vi "will_heading_hit_obstacles.vi"(8 "Distance to check (m)":dbl, 9 "Heading":dbl, 10 "Boat Location":T1 {"North" format="%#_10f"; "East" format="%#_8f"}, 11 "Obstacle array":refnum<class "Obstacle.lvclass">[](array[class])) -> (3 "Will boat hit any obstacles?":bool)   [LabVIEW 2013]
uses:
  Obstacle.lvclass
  Data/TypeDefs/UTM Location.ctl
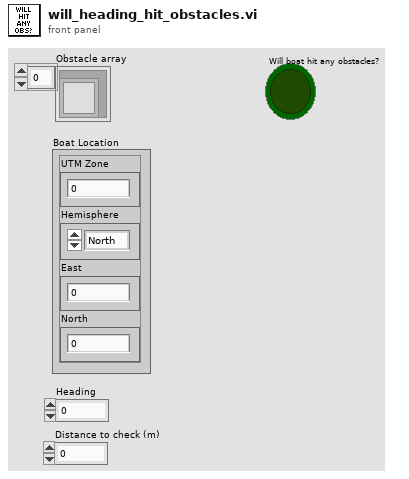
[diagram p1: front panel]
types:
  T1 = typedef "UTM Location.ctl" = cluster{"UTM Zone":dbl, "Hemisphere":enum16{"North", "South"}, "East":dbl, "North":dbl}
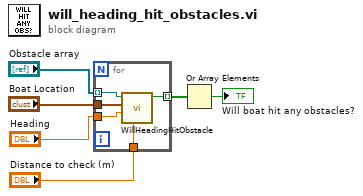
[diagram p0: block diagram]
diagram:
  n1 = for {
    tunnel: "Obstacle array" -> [w11] mode=indexing
    tunnel: [w10] -> w6 mode=indexing
    tunnel: "Boat Location" -> [w9]
    tunnel: "Heading" -> [w8]
    tunnel: "Distance to check (m)" -> [w7]
    n2 = call "WillHeadingHitObstacle.vi"("Distance to check (m)"=w7, "Heading"=w8, "Boat"=w9, "Obstacle.lvclass"=w11) -> ("Any intersecting obstacles?"=w10:bool)  [unwired: 6 in, 1 out]
  }
  n3 = Or Array Elements(Boolean array=w6) -> (logical OR=→"Will boat hit any obstacles?":bool)
